vi "Formula_Node_Ejercicio.vi"() -> ()   [LabVIEW 2020]
panel:
  out "XY Graph":cluster{dbl[], dbl[]}(graph)
  out "Waveform Graph":dbl[](graph)
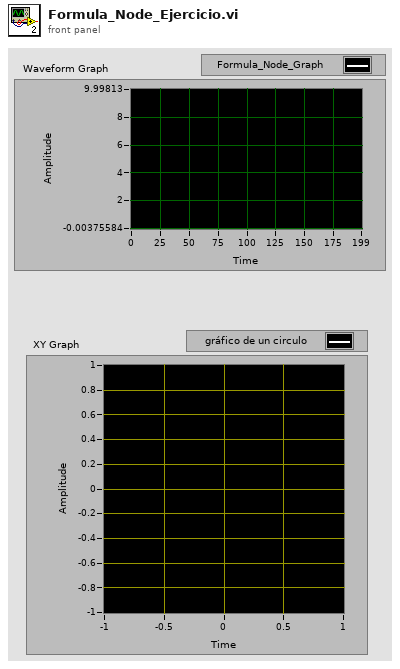
[diagram p1: front panel]
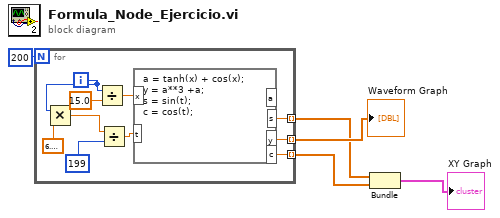
[diagram p0: block diagram]
diagram:
  n1 = for {
    N: 200 -> [_]
    tunnel: [w13] -> w4 mode=indexing
    tunnel: [w10] -> w3 mode=indexing
    tunnel: [w9] -> w2 mode=indexing
    i -> [w8]
    n2 = Multiply(x=w8, y=6.283185307179586) -> (x*y=w6:dbl)
    n3 = Divide(x=w8, y=15.0) -> (x/y=w14:dbl)
    n4 = Divide(x=w6, y=199) -> (x/y=w11:dbl)
    n5 = formula code="a = tanh(x) + cos(x);\ny = a**3 +a;\ns = sin(t);\nc = cos(t);"("x"=w14, "t"=w11) -> ("y"=w13:dbl, "s"=w10:dbl, "c"=w9:dbl)  [unwired: 1 out]
  }
  "Waveform Graph" <- w4
  n6 = Bundle(w3, w2) -> (→"XY Graph":cluster{dbl[], dbl[]})  [unwired: 1 in]
